vi "Quiz2_try.vi"() -> ()   [LabVIEW 2020]
panel:
  in  "X":dbl
  in  "Y":dbl
  out "Devide by Zero":bool
  out "X / Y":dbl
  out "X + Y":dbl
  out "X - Y":dbl
  out "X x Y":dbl
  out "length":i32
  out "concatenated string":string
  out "decimal integer string":string
  out "error out":errorcluster
  in  "Send to Server":bool
  out "error out 2":errorcluster
  out "error out 3":errorcluster
  out "error out 4":errorcluster
  # "Client"
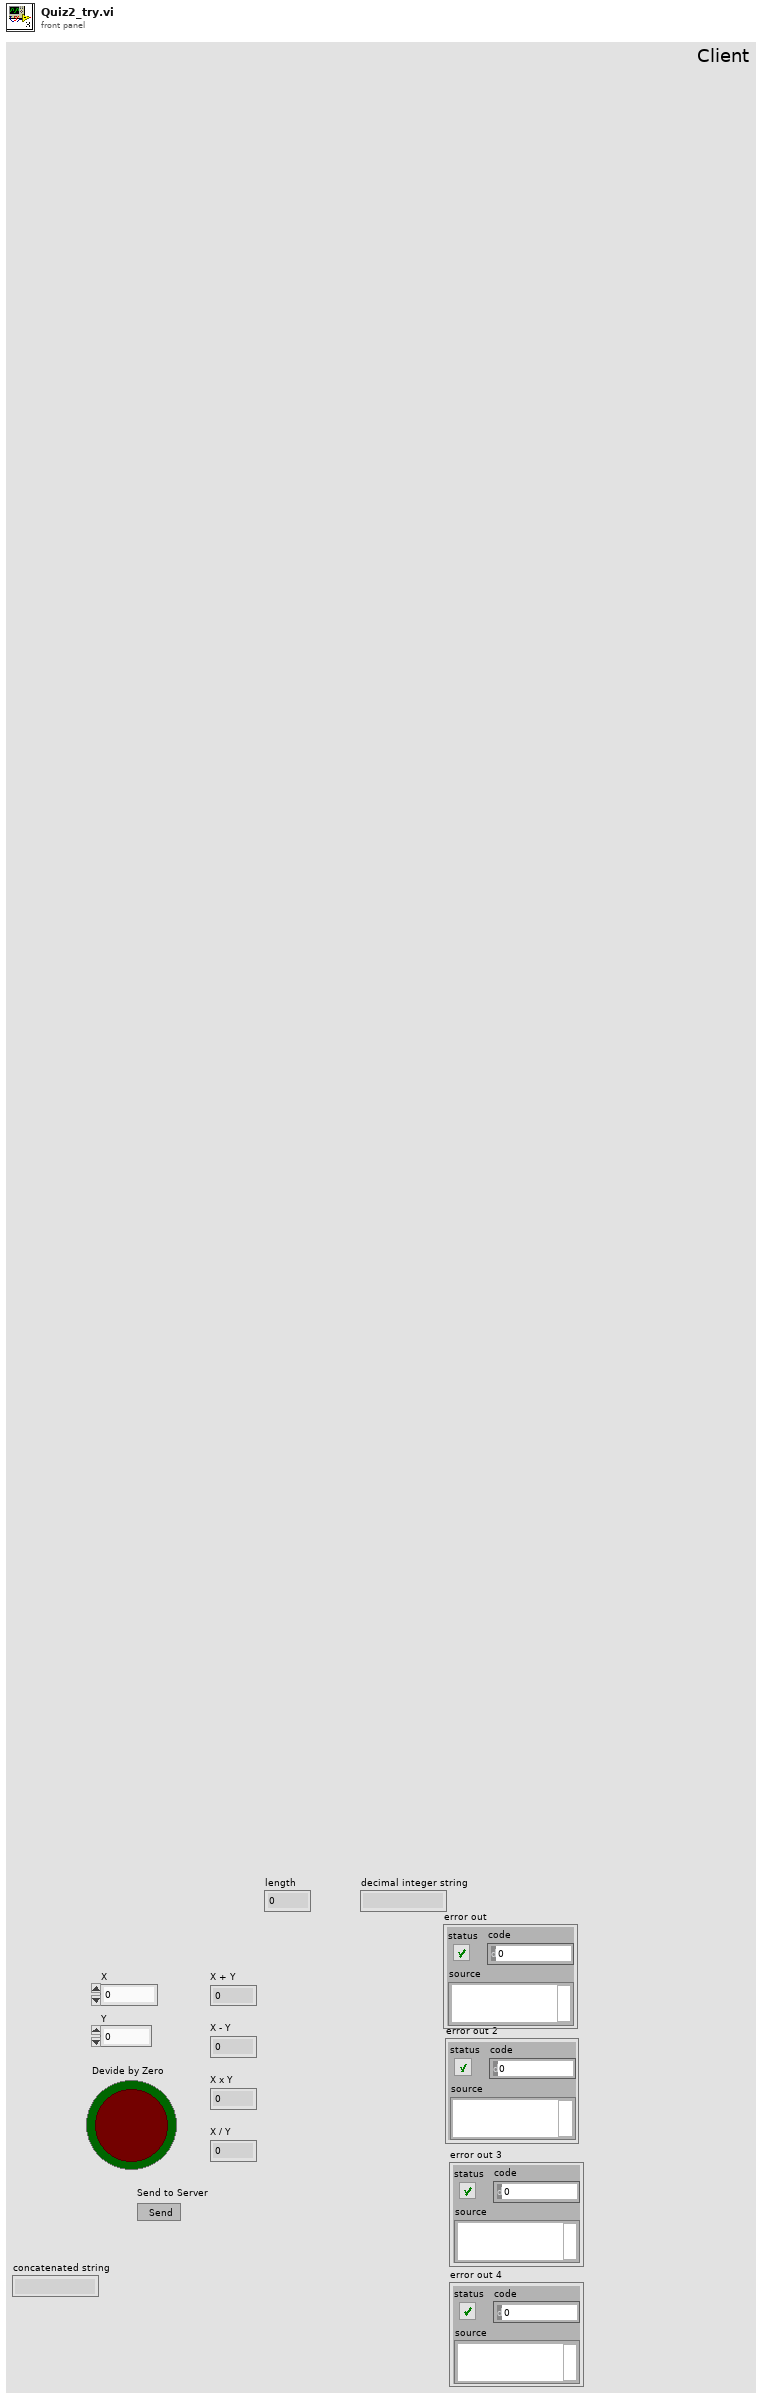
[diagram p1: front panel]
types:
  T1 = enum8{"Enabled", "Disabled", "Disabled and Grayed Out"}
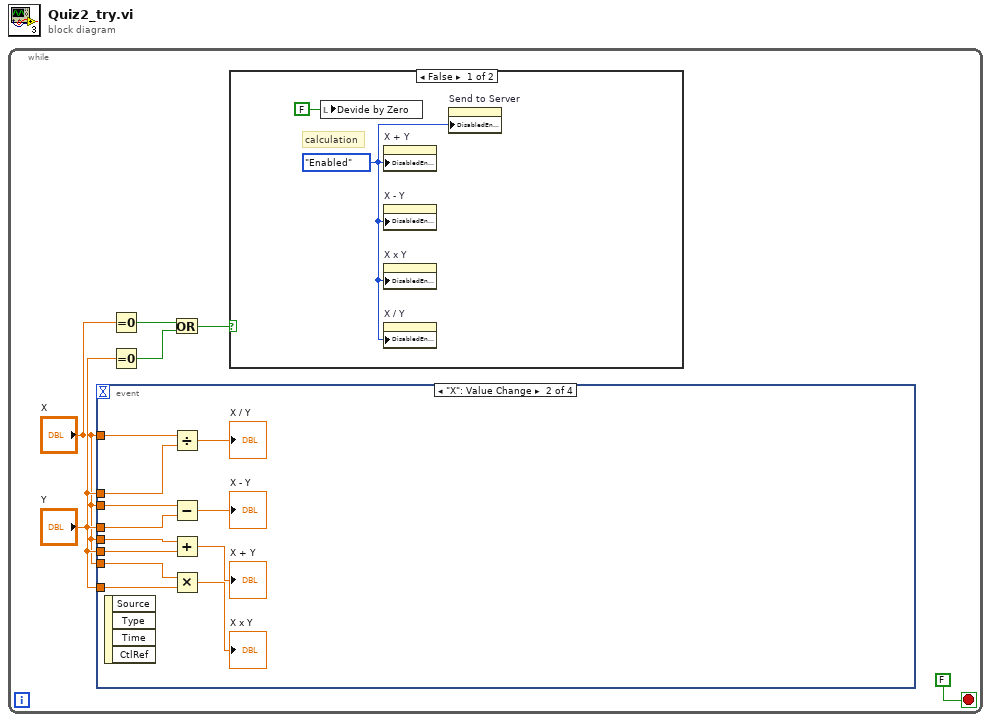
[diagram p0: block diagram]
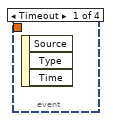
[diagram p2: hidden frame]
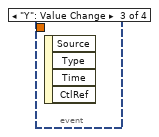
[diagram p3: hidden frame]
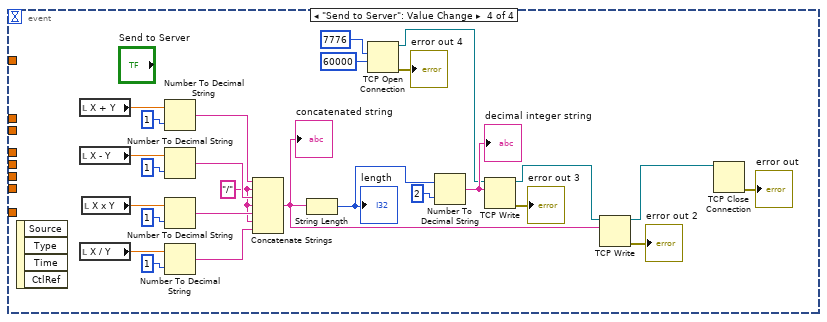
[diagram p4: hidden frame]
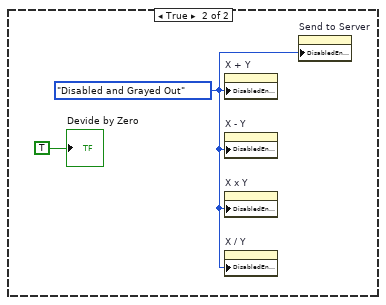
[diagram p5: hidden frame]
diagram:
  n1 = while {
    stop <- FALSE stop-if-true
    n2 = event shown="[1] \"X\": Value Change" {
      selector: _ -> [_ _ _ _]
      dyn-events: _ -> [_ _ _ _]
      timeout: _ -> [_ _ _ _]
      tunnel: "Y" -> [_ w14 _ _]
      tunnel: "X" -> [_ w13 _ _]
      tunnel: "Y" -> [_ w12 _ _]
      tunnel: "X" -> [_ w11 _ _]
      tunnel: "Y" -> [_ w10 _ _]
      tunnel: "X" -> [_ w9 _ _]
      tunnel: "Y" -> [_ w8 _ _]
      tunnel: "X" -> [_ w7 _ _]
      event Timeout {
        n3 = event-data() -> ()  [unwired: 1 in, 3 out]
      }
      event "X": Value Change {
        n4 = event-data() -> ()  [unwired: 1 in, 4 out]
        n5 = Divide(x=w7, y=w8) -> (x/y=→"X / Y":dbl)
        n6 = Subtract(x=w11, y=w12) -> (x-y=→"X - Y":dbl)
        n7 = Add(x=w9, y=w10) -> (x+y=→"X + Y":dbl)
        n8 = Multiply(x=w13, y=w14) -> (x*y=→"X x Y":dbl)
      }
      event "Y": Value Change {
        n9 = event-data() -> ()  [unwired: 1 in, 4 out]
      }
      event "Send to Server": Value Change {
        w19 = "/" ("string")
        n10 = event-data() -> ()  [unwired: 1 in, 4 out]
        n11 = local read "X + Y"() -> (w37:dbl)
        n12 = local read "X - Y"() -> (w40:dbl)
        n13 = local read "X / Y"() -> (w38:dbl)
        n14 = local read "X x Y"() -> (w39:dbl)
        n15 = Number To Decimal String(number=w37, width (-)=i16 1) -> (decimal integer string=w41:string)
        n16 = Number To Decimal String(number=w40, width (-)=i16 1) -> (decimal integer string=w42:string)
        n17 = Number To Decimal String(number=w39, width (-)=i16 1) -> (decimal integer string=w43:string)
        n18 = Number To Decimal String(number=w38, width (-)=i16 1) -> (decimal integer string=w44:string)
        n19 = Concatenate Strings(w41, w19, w42, w19, w43, w19, w44) -> (w31:string)
        "concatenated string" <- w31
        n20 = String Length(string=w31) -> (length=w33:i32)
        "length" <- w33
        n21 = TCP Open Connection(remote port or service name=u16 7776, timeout ms (60000)=60000) -> (connection ID=w28:refnum<k5>, error out=→"error out 4":errorcluster)  [unwired: 3 in]
        n22 = Number To Decimal String(number=w33, width (-)=i16 2) -> (decimal integer string=w30:string)
        "decimal integer string" <- w30
        n23 = TCP Write(connection ID=w28, data in=w30) -> (connection ID out=w29:refnum<k5>, error out=→"error out 3":errorcluster)  [unwired: 2 in, 1 out]
        n24 = TCP Write(connection ID=w29, data in=w31) -> (connection ID out=w32:refnum<k5>, error out=→"error out 2":errorcluster)  [unwired: 2 in, 1 out]
        n25 = TCP Close Connection(connection ID=w32) -> (error out=→"error out":errorcluster)  [unwired: 2 in, 1 out]
      }
    }
    n26 = Equal To 0?(x="X") -> (x = 0?=w5:bool)
    n27 = Equal To 0?(x="Y") -> (x = 0?=w4:bool)
    n28 = Or(x=w5, y=w4) -> (x .or. y?=w3:bool)
    n29 = case shown="False" w3 {
      frame False {
        w46 = T1."Enabled" ("Disabled")
        # "calculation"
        n30 = local write "Devide by Zero"(FALSE ("Devide by Zero")) -> ()
        n31 = property on="X + Y" class="DigNum (strict)"("DisabledEnum"=w46) -> ()  [unwired: 2 in, 2 out]
        n32 = property on="X - Y" class="DigNum (strict)"("DisabledEnum"=w46) -> ()  [unwired: 2 in, 2 out]
        n33 = property on="X x Y" class="DigNum (strict)"("DisabledEnum"=w46) -> ()  [unwired: 2 in, 2 out]
        n34 = property on="X / Y" class="DigNum (strict)"("DisabledEnum"=w46) -> ()  [unwired: 2 in, 2 out]
        n35 = property on="Send to Server" class="Bool"("DisabledEnum"=w46) -> ()  [unwired: 2 in, 2 out]
      }
      frame True {
        w48 = T1."Disabled and Grayed Out" ("Disabled")
        n36 = property on="X + Y" class="DigNum (strict)"("DisabledEnum"=w48) -> ()  [unwired: 2 in, 2 out]
        n37 = property on="X - Y" class="DigNum (strict)"("DisabledEnum"=w48) -> ()  [unwired: 2 in, 2 out]
        n38 = property on="X x Y" class="DigNum (strict)"("DisabledEnum"=w48) -> ()  [unwired: 2 in, 2 out]
        n39 = property on="X / Y" class="DigNum (strict)"("DisabledEnum"=w48) -> ()  [unwired: 2 in, 2 out]
        n40 = property on="Send to Server" class="Bool"("DisabledEnum"=w48) -> ()  [unwired: 2 in, 2 out]
        "Devide by Zero" <- TRUE ("Devide by Zero")
      }
    }
  }
